vi "개별쓰기(Main).vi"() -> ()   [LabVIEW 2014]
panel:
  out "Error Code":string
  in  "데이터":u16[](array[numeric])=[13106, 13104] format="%.0x"
  in  "변수이름 배열":string[](array[string])=["%DW0000", "%DW0002"]
  out "에러 출력":errorcluster
  in  "주소":string="192.168.0.10"
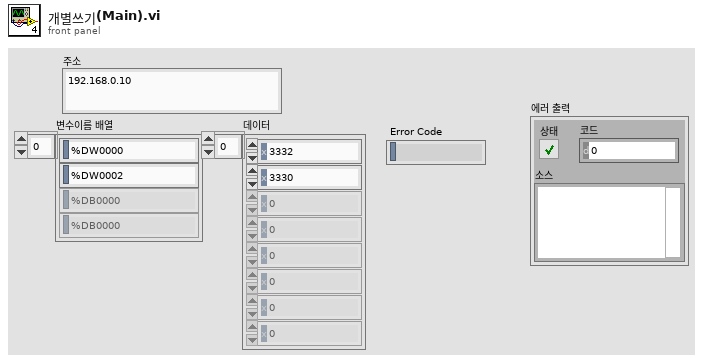
[diagram p1: front panel]
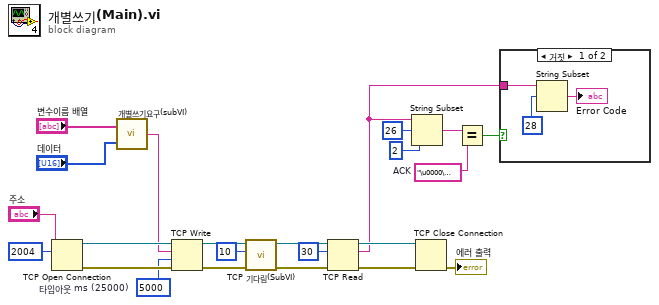
[diagram p0: block diagram]
diagram:
  w3 = "\u0000\u0000"  # ACK
  w10 = 5000  # 타임아웃 ms (25000)
  n1 = TCP Open Connection(address="주소", remote port or service name=u16 2004 ("원격 포트 또는 서비스 이름")) -> (connection ID=w21:refnum<k5>, error out=w20:errorcluster)  [unwired: 3 in]
  n2 = call "개별쓰기요구(subVI).vi"("데이터"="데이터", "변수이름 배열"="변수이름 배열") -> ("개별쓰기"=w9:string)
  n3 = TCP Write(connection ID=w21, data in=w9, error in (no error)=w20, 9:w10) -> (connection ID out=w15:refnum<k5>, error out=w13:errorcluster)  [unwired: 1 out]
  n4 = call "TCP 기다림(SubVI).vi"("error in"=w13, "기다림(ms)"=u32 10, "TCP 네트워크 연결 입력"=w15) -> ("error out"=w12:errorcluster, "TCP 네트워크 연결 출력"=w14:refnum<k5>)  [unwired: 7 in]
  n5 = TCP Read(connection ID=w14, bytes to read=30 ("읽을 바이트"), error in (no error)=w12) -> (connection ID out=w19:refnum<k5>, data out=w1:string, error out=w18:errorcluster)  [unwired: 2 in]
  n6 = String Subset(string=w1, offset (0)=26 ("오프셋(0)"), length (rest)=2 ("길이(나머지)")) -> (substring=w4:string)
  n7 = TCP Close Connection(connection ID=w19, error in (no error)=w18) -> (error out=→"에러 출력":errorcluster)  [unwired: 1 in, 1 out]
  n8 = Equal?(x=w4, y=w3) -> (x = y?=w2:bool)
  n9 = case shown="거짓" w2 {
    tunnel: w1 -> [w26 _]
    frame False {
      n10 = String Subset(string=w26, offset (0)=28 ("오프셋(0)")) -> (substring=→"Error Code":string)  [unwired: 1 in]
    }
    frame True {
    }
  }
